vi "MVi Relative Path 2 Me.vi"(5 "Relative Path":string) -> (1 "Appended Dir":path, 2 "MyDir":path)   [LabVIEW 2017]
panel:
  # "Input Parameters"
  # "Output Parameters"
  # "VI Description:\nThis VI is created to Grab a image from imaging device."
  # ":: MVI Framework V1.0 ::\nAuthor:Gaoke Yang\nEmail: gaoke.yang@yahoo.com\nWeb: www.mvicontrol.com\nCopyright (C) 2015, MVI Technologies All Rights Reserved"
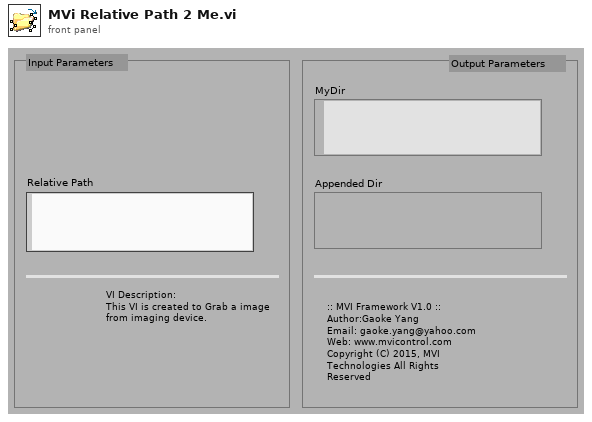
[diagram p1: front panel]
types:
  T1 = enum32{"invalid app kind", "Development System", "Run Time System", "Student Edition", "Embedded LabVIEW", "Evaluation", "Custom"}
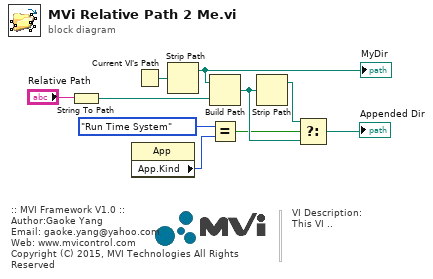
[diagram p0: block diagram]
diagram:
  # "VI Description:\nThis VI .."
  # ":: MVI Framework V1.0 ::\nAuthor:Gaoke Yang\nEmail: gaoke.yang@yahoo.com\nWeb: www.mvicontrol.com\nCopyright (C) 2015, MVI Technologies All Rights Reserved"
  n1 = String To Path(string="Relative Path") -> (path=w2:path)
  n2 = property class="App"() -> ("App.Kind"=w8:T1)  [unwired: 2 in, 2 out]
  n3 = Current VI's Path() -> (path=w5:path)
  n4 = Strip Path(path=w5) -> (stripped path=w3:path)  [unwired: 1 out]
  "MyDir" <- w3
  n5 = Build Path(base path=w3, name or relative path=w2) -> (appended path=w9:path)
  n6 = Equal?(x=T1."Run Time System" ("Application:Kind"), y=w8) -> (x = y?=w6:bool)
  n7 = Strip Path(path=w9) -> (stripped path=w10:path)  [unwired: 1 out]
  n8 = Select(t=w10, s=w6, f=w9) -> (s? t:f=→"Appended Dir":path)
